vi "Q to Euler.vi"(6 "value":T1) -> (0 "Roll":dbl, 1 "Yaw":dbl, 2 "Waveform Chart":cluster{"Yaw":dbl, "Pitch":dbl, "Roll":dbl}(graph), 3 "Pitch":dbl)   [LabVIEW 2015]
panel:
  # "This VI converts quanternion to Euler angles.\nnotice that the first three input variables (qx,qy,qz) represents the vector element,\nwhile the forth (qw) is the scalar element."
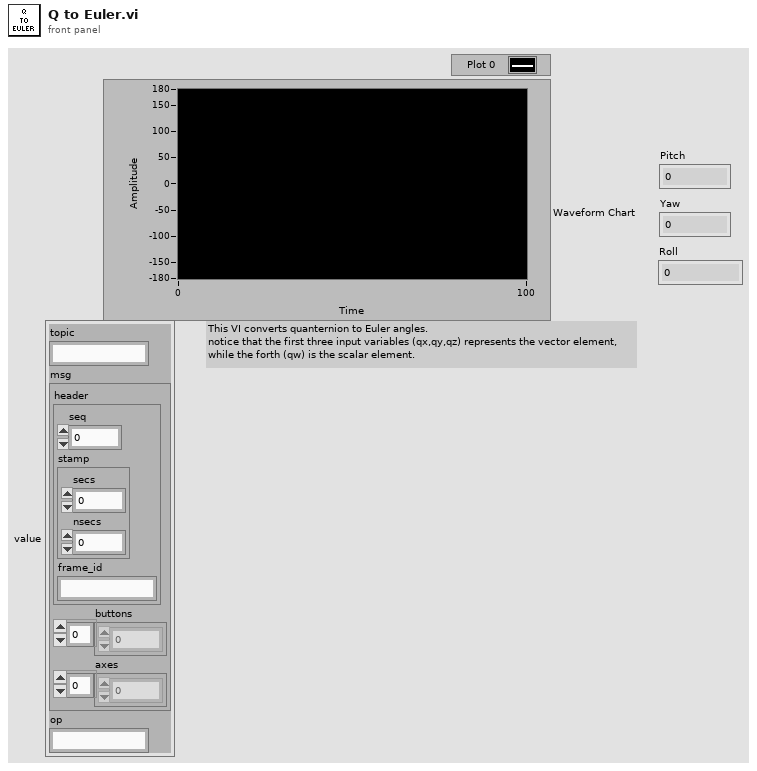
[diagram p1: front panel]
types:
  T1 = cluster{"topic":string, "msg":cluster{"header":cluster{"seq":u32, "stamp":cluster{"secs":u32, "nsecs":i32}, "frame_id":string}, "buttons":i32[], "axes":sgl[]}, "op":string}
  T2 = cluster{"header":cluster{"seq":u32, "stamp":cluster{"secs":u32, "nsecs":i32}, "frame_id":string}, "buttons":i32[], "axes":sgl[]}
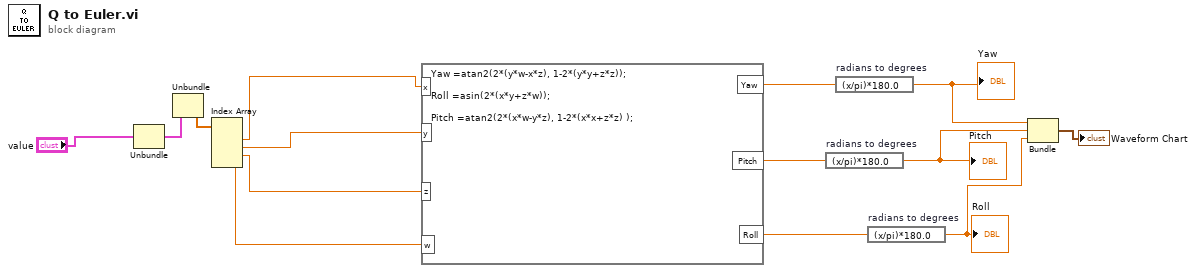
[diagram p0: block diagram]
diagram:
  n1 = Unbundle("value") -> ("msg"=w11:T2)  [unwired: 2 out]
  n2 = Unbundle(w11) -> ("axes"=w10:sgl[])  [unwired: 2 out]
  n3 = Index Array(array=w10) -> (element #1=w9:sgl, element #2=w8:sgl, element #3=w7:sgl, element #4=w6:sgl)  [unwired: 4 in]
  n4 = formula code="Yaw =atan2(2*(y*w-x*z),\t1-2*(y*y+z*z));\n\nRoll =asin(2*(x*y+z*w));\n\nPitch =atan2(2*(x*w-y*z), 1-2*(x*x+z*z) );"("x"=w9, "y"=w8, "z"=w7, "w"=w6) -> ("Yaw"=w14:dbl, "Pitch"=w13:dbl, "Roll"=w12:dbl)
  n5 = expression code="(x/pi)*180.0" "radians to degrees"(w13) -> (w4:dbl)
  "Pitch" <- w4
  n6 = expression code="(x/pi)*180.0" "radians to degrees"(w14) -> (w5:dbl)
  "Yaw" <- w5
  n7 = expression code="(x/pi)*180.0" "radians to degrees"(w12) -> (w3:dbl)
  "Roll" <- w3
  n8 = Bundle("Yaw"=w5, "Pitch"=w4, "Roll"=w3) -> (→"Waveform Chart":cluster{"Yaw":dbl, "Pitch":dbl, "Roll":dbl})  [unwired: 1 in]
